vi "Write Movie Name.vi"(8 "error in (no error)":errorcluster, 10 "Movie Name":string, 11 "Adam Sandler in":refnum<class "Adam Sandler.lvclass">) -> (0 "error out":errorcluster, 3 "Adam Sandler out":refnum<class "Adam Sandler.lvclass">)   [LabVIEW 2019, in "Adam Sandler.lvclass"]
uses:
  Adam Sandler.lvclass
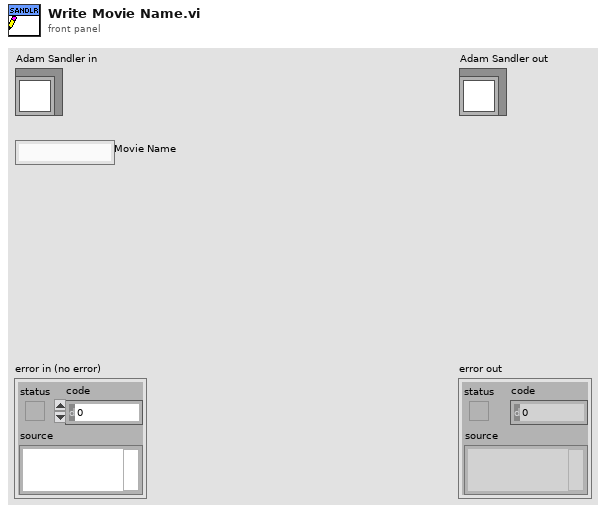
[diagram p1: front panel]
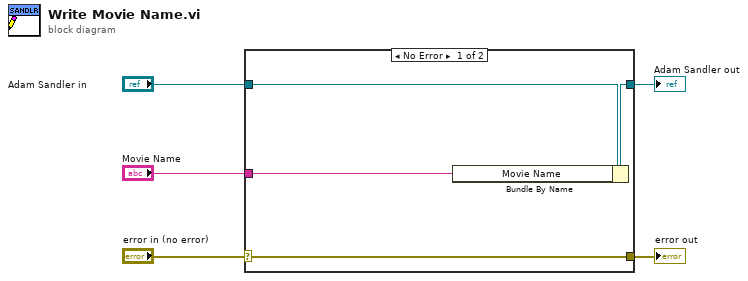
[diagram p0: block diagram]
diagram:
  n1 = case shown="No Error" "error in (no error)" {
    selector: "error in (no error)" -> [w9 w10]
    tunnel: [w9 w10] -> w4
    tunnel: [w7 w11] -> w2
    tunnel: "Adam Sandler in" -> [w8 w11]
    tunnel: "Movie Name" -> [w6 _]
    frame No Error {
      n2 = Bundle By Name(cluster=w8, "Movie Name"=w6) -> (w7:refnum<class "Adam Sandler.lvclass">)
    }
    frame Error {
    }
  }
  "error out" <- w4
  "Adam Sandler out" <- w2
